vi "_test_ArrangeVI (VI).vi"() -> ()   [LabVIEW 2020]
panel:
  in  "save VI":bool
  in  "Show FP":bool
  out "error out":errorcluster
  in  "FP":bool
  in  "VI Path":path=path "C:/Users/Administrator/Desktop/Azdo/emea-aim-664-instrument-driver-1204/src/AIM664LV.lvlib"
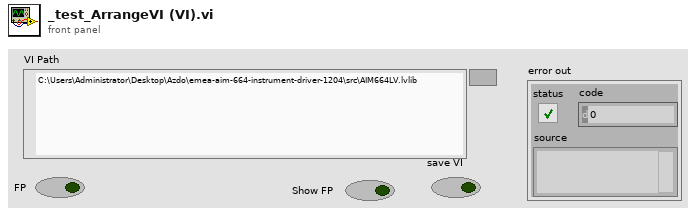
[diagram p1: front panel]
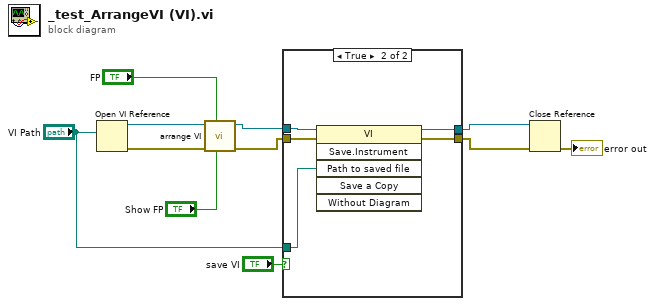
[diagram p0: block diagram]
diagram:
  n1 = Open VI Reference(vi path="VI Path") -> (vi reference=w11:refnum<vi>, error out=w10:errorcluster)  [unwired: 5 in]
  n2 = call "arrange VI.vi"("Show FP (F)"="Show FP", "FP (T)"="FP", "error in"=w10, "VI in"=w11) -> ("error out"=w5:errorcluster, "VI out"=w6:refnum<vi>)  [unwired: 6 in]
  n3 = case shown="True" "save VI" {
    tunnel: w6 -> [w13 w18]
    tunnel: [w13 w15] -> w4
    tunnel: w5 -> [w12 w17]
    tunnel: [w12 w16] -> w3
    tunnel: "VI Path" -> [_ w14]
    frame False {
    }
    frame True {
      n4 = invoke class="VI" method="Save.Instrument"(reference=w18, error in=w17, "Path to saved file"=w14) -> (reference out=w15:refnum<vi>, error out=w16:errorcluster)  [unwired: 3 in, 4 out]
    }
  }
  n5 = Close Reference(reference=w4, error in (no error)=w3) -> (error out=→"error out":errorcluster)
